vi "Parse Timestamp Array.vi"(6 "Seperator":string=",", 8 "error in":errorcluster, 9 "Input <JSON>":string, 10 "csv string":string, 11 "Simple CSV Parser in":refnum<class "Simple CSV Parser.lvclass">) -> (0 "error out":errorcluster, 2 "Timestamp Array":timestamp[](array[timestamp]) format="%<%x %.3X>T", 3 "Simple CSV Parser out":refnum<class "Simple CSV Parser.lvclass">)   [LabVIEW 2020, in "Simple CSV Parser.lvclass"]
uses:
  Simple CSV Parser.lvclass
  Simple CSV Parser.lvclass/Simple CSV Parser.ctl
  dee25020-1756-461a-ae13-2f1165168e5a.vi
  4bb66f33-81c4-4fca-9d50-ff929125331a.vi
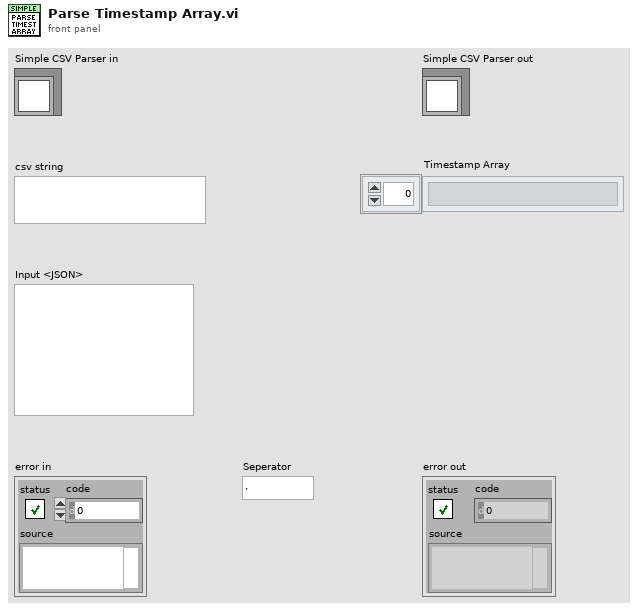
[diagram p1: front panel]
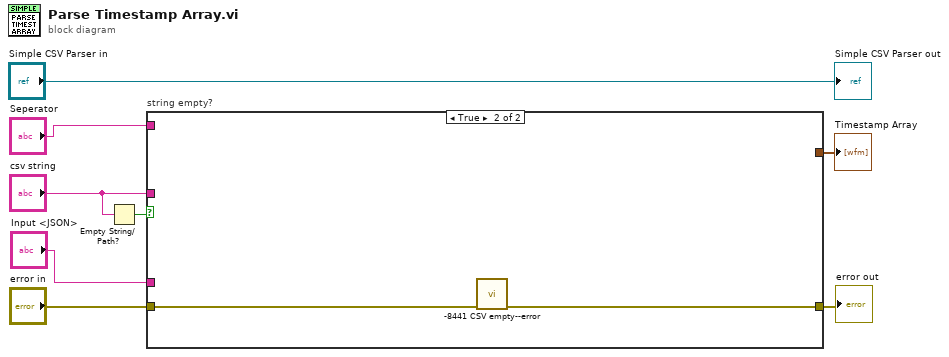
[diagram p0: block diagram]
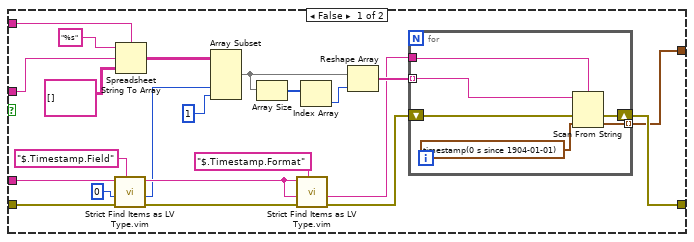
[diagram p2: hidden frame]
diagram:
  n1 = Empty String/Path?(string/path="csv string") -> (empty?=w2:bool)
  n2 = case "string empty?" shown="True" w2 {
    tunnel: "error in" -> [w22 w38]
    tunnel: [w21 w37] -> w6
    tunnel: [w20 _] -> w5
    tunnel: "Seperator" -> [w19 _]
    tunnel: "csv string" -> [w18 _]
    tunnel: "Input <JSON>" -> [w13 _]
    frame False {
      n3 = call "Strict Find Items as LV Type.vim"("$Path or Item Name"="$.Timestamp.Field", "error in"=w22, "Data Type and Default Value"=0, "<JSON>"=w13) -> ("error out"=w14:errorcluster, "Data out"=w9:i32, "<JSON> dup"=w12:string)  [unwired: 5 in]
      n4 = Spreadsheet String To Array(delimiter (Tab)=w19, format string="%s", spreadsheet string=w18, array type (2D Dbl)=string[][] []) -> (array=w27:string[][])
      n5 = Array Subset(array=w27, index (col)=w9, length (col)=1 ("length")) -> (w25:string[][])  [unwired: 2 in]
      n6 = Array Size(array=w25) -> (size(s)=w26:i32[])
      n7 = call "Strict Find Items as LV Type.vim"("$Path or Item Name"="$.Timestamp.Format", "error in"=w14, "Data Type and Default Value"=w12, "<JSON>"=w12) -> ("error out"=w17:errorcluster, "Data out"=w15:string)  [unwired: 5 in, 1 out]
      n8 = Index Array(array=w26) -> (element=w24:i32)  [unwired: 1 in]
      n9 = Reshape Array(w25, w24) -> (w23:string[])
      n10 = for {
        tunnel: w15 -> [w36]
        shift-right: [w34] -> w21
        shift-left: w17 -> [w35]
        tunnel: w23 -> [w33] mode=indexing
        tunnel: [w32] -> w20 mode=indexing
        n11 = Scan From String(format string=w36, input string=w33, error in=w35, default 1=timestamp(0 s since 1904-01-01) ("Time Stamp")) -> (error out=w34:errorcluster, output 1=w32:timestamp)  [unwired: 1 in, 2 out]
      }
    }
    frame True {
      n12 = call "-8441 CSV empty--error.vi"("error in"=w38) -> ("error out"=w37:errorcluster)  [unwired: 10 in]
    }
  }
  "error out" <- w6
  "Timestamp Array" <- w5
  "Simple CSV Parser out" <- "Simple CSV Parser in"
